vi "NI VeriStand - Set Aliases.vi"(7 "Runtime Alias Folder Name":string, 8 "Error in":errorcluster, 9 "Alias Names":string[](array[string]), 10 "Referenced Channels":string[](array[string]), 11 "Runtime Configuration Ref in":refnum<k39>) -> (0 "Error out":errorcluster, 3 "Runtime Configuration Ref out":refnum<k39>, 5 "Success":bool)   [LabVIEW 2025, in "Runtime Configuration File API.lvlib"]
uses:
  Runtime Configuration File API.lvlib
  C:/NetCoreDLL/NationalInstruments.VeriStand.SystemDefinitionAPI.dll
  NetCoreDLL/NationalInstruments.VeriStand.SystemDefinitionAPI.dll
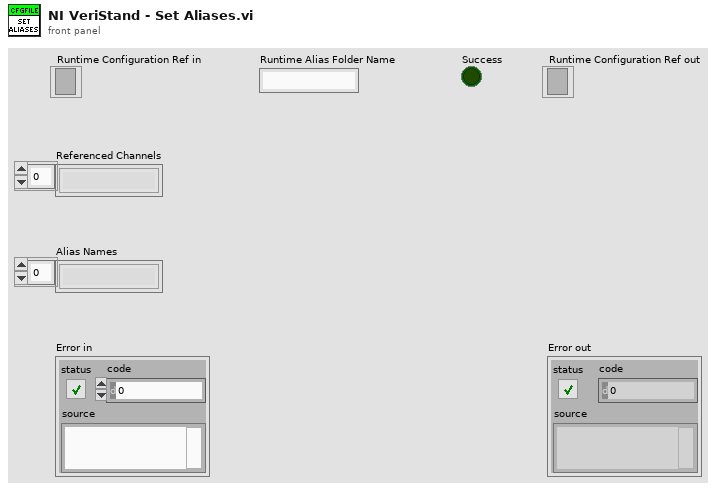
[diagram p1: front panel]
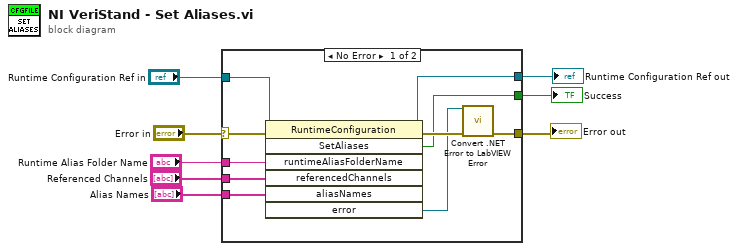
[diagram p0: block diagram]
diagram:
  n1 = case shown="No Error" "Error in" {
    selector: "Error in" -> [w18 w19]
    tunnel: "Runtime Configuration Ref in" -> [w15 _]
    tunnel: "Runtime Alias Folder Name" -> [w14 _]
    tunnel: "Referenced Channels" -> [w13 _]
    tunnel: "Alias Names" -> [w12 _]
    tunnel: [w11 _] -> w2
    tunnel: [w16 w19] -> w8
    tunnel: [w10 _] -> w1
    frame No Error {
      n2 = invoke class="RuntimeConfiguration" method="SetAliases"(reference=w15, error in=w18, "runtimeAliasFolderName"=w14, "referencedChannels"=w13, "aliasNames"=w12) -> (reference out=w11:refnum<k39>, error out=w17:errorcluster, "SetAliases"=w10:bool, "error"=w9:refnum<k39>)  [unwired: 2 in, 3 out]
      n3 = call "Convert .NET Error to LabVIEW Error.vi"("error in"=w17, "NationalInstruments.VeriStand.Error"=w9) -> ("error out"=w16:errorcluster)  [unwired: 9 in]
    }
    frame Error {
    }
  }
  "Runtime Configuration Ref out" <- w2
  "Error out" <- w8
  "Success" <- w1
